vi "FGV_DataLoggerControl.vi"(7 "Actions":T1, 8 "Error In":errorcluster, 9 "Value":i32, 11 "VISA Refnum in":refnum<visa-resource-name>="COM1") -> (0 "Error Out":errorcluster, 1 "read buffer":string, 3 "VISA Refnum out":refnum<visa-resource-name>="COM1")   [LabVIEW 2014]
uses:
  Typedef_DataLogger_Actions.ctl
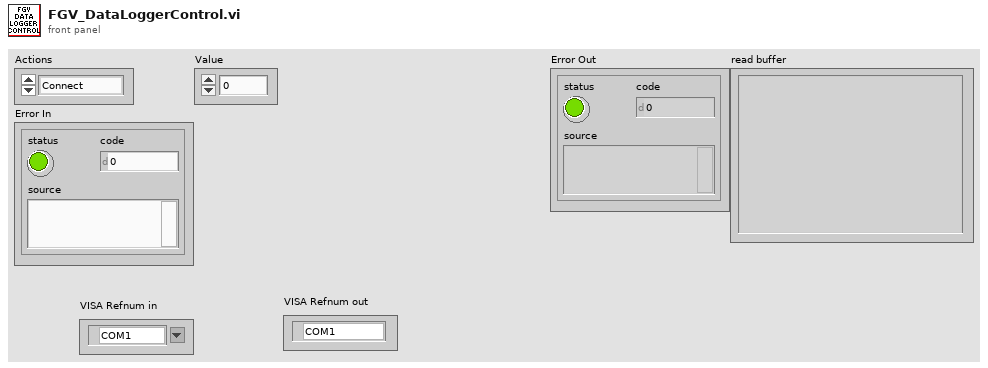
[diagram p1: front panel]
types:
  T1 = typedef "Typedef_DataLogger_Actions.ctl" = enum16{"Connect", "Disconnect", "Get Reading", "Set Offset", "Get Offset", "Set Time Step", "Get Time Step", "Save Settings", "Disable Readings", "Enable Readings"}
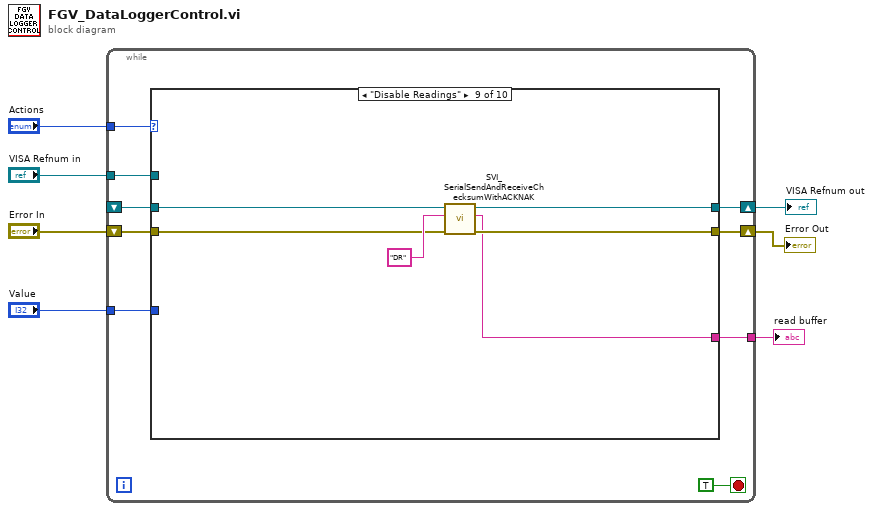
[diagram p0: block diagram]
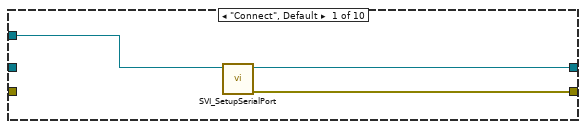
[diagram p2: hidden frame]
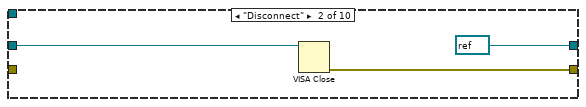
[diagram p3: hidden frame]
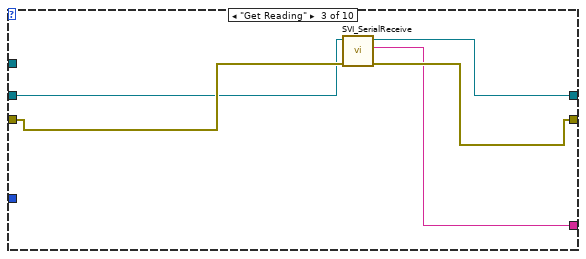
[diagram p4: hidden frame]
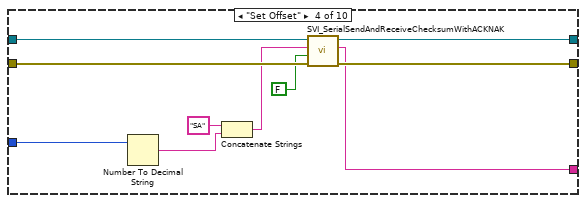
[diagram p5: hidden frame]
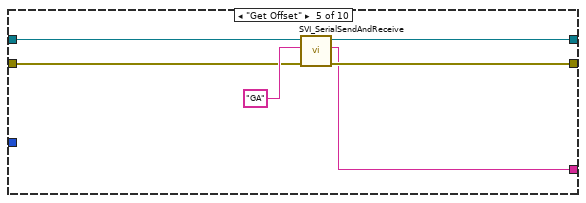
[diagram p6: hidden frame]
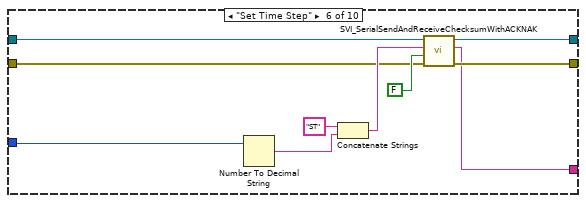
[diagram p7: hidden frame]
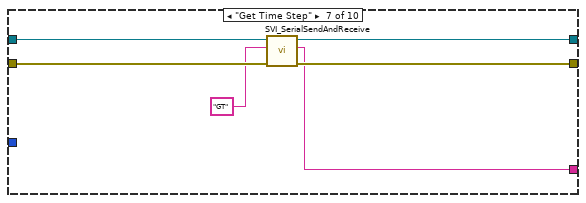
[diagram p8: hidden frame]
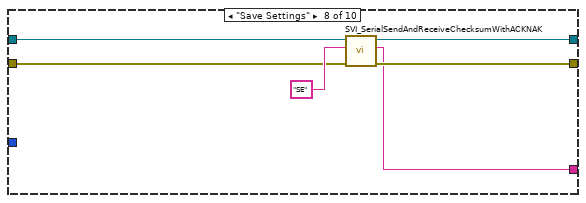
[diagram p9: hidden frame]
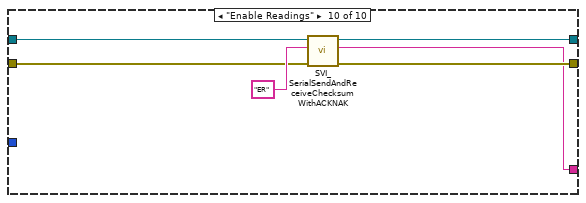
[diagram p10: hidden frame]
diagram:
  n1 = while {
    tunnel: "Actions" -> [w15]
    tunnel: "VISA Refnum in" -> [w14]
    shift-right: [w13] -> w3
    shift-left: _ -> [w11]
    shift-right: [w12] -> w5
    shift-left: "Error In" -> [w10]
    tunnel: "Value" -> [w9]
    tunnel: [w8] -> w1
    stop <- TRUE stop-if-true
    n2 = case shown="\"Disable Readings\"" w15 {
      tunnel: w14 -> [w19 _ _ _ _ _ _ _ _ _]
      tunnel: [w18 refnum<visa-resource-name> refnum ("VISA resource name out") w24 w33 w41 w46 w58 w63 w68 w74] -> w13
      tunnel: [w17 w22 w25 w34 w42 w47 w59 w64 w67 w73] -> w12
      tunnel: w11 -> [_ w20 w26 w36 w40 w48 w56 w62 w69 w75]
      tunnel: w10 -> [_ _ w27 w35 w39 w49 w57 w61 w70 w76]
      tunnel: w9 -> [_ _ _ w31 _ w45 _ _ _ _]
      tunnel: [_ _ w23 w28 w38 w44 w54 w60 w66 w72] -> w8
      frame "Connect", Default {
        n3 = call "SVI_SetupSerialPort.vi"("VISA Refnum in"=w19) -> ("error out"=w17:errorcluster, "VISA Refnum out"=w18:refnum<visa-resource-name>)  [unwired: 9 in]
      }
      frame "Disconnect" {
        n4 = VISA Close(VISA resource name=w20) -> (error out=w22:errorcluster)  [unwired: 1 in]
      }
      frame "Get Reading" {
        n5 = call "SVI_SerialReceive.vi"("error in (no error)"=w27, "VISA Refnum in"=w26) -> ("error out"=w25:errorcluster, "read buffer"=w23:string, "VISA resource name out"=w24:refnum<visa-resource-name>)  [unwired: 7 in]
      }
      frame "Set Offset" {
        n6 = Number To Decimal String(number=w31) -> (decimal integer string=w29:string)  [unwired: 1 in]
        n7 = Concatenate Strings("SA" ("Command"), w29) -> (w30:string)
        n8 = call "SVI_SerialSendAndReceiveChecksumWithACKNAK.vi"("error in (no error)"=w35, "Send Checksum"=FALSE, "Command"=w30, "VISA Refnum in"=w36) -> ("error out"=w34:errorcluster, "Received"=w28:string, "VISA resource name out"=w33:refnum<visa-resource-name>)  [unwired: 5 in]
      }
      frame "Get Offset" {
        n9 = call "SVI_SerialSendAndReceive.vi"("error in (no error)"=w39, "Command"="GA", "VISA Refnum in"=w40) -> ("error out"=w42:errorcluster, "read buffer"=w38:string, "VISA resource name out"=w41:refnum<visa-resource-name>)  [unwired: 6 in]
      }
      frame "Set Time Step" {
        n10 = Number To Decimal String(number=w45) -> (decimal integer string=w50:string)  [unwired: 1 in]
        n11 = Concatenate Strings("ST" ("Command"), w50) -> (w51:string)
        n12 = call "SVI_SerialSendAndReceiveChecksumWithACKNAK.vi"("error in (no error)"=w49, "Send Checksum"=FALSE, "Command"=w51, "VISA Refnum in"=w48) -> ("error out"=w47:errorcluster, "Received"=w44:string, "VISA resource name out"=w46:refnum<visa-resource-name>)  [unwired: 5 in]
      }
      frame "Get Time Step" {
        n13 = call "SVI_SerialSendAndReceive.vi"("error in (no error)"=w57, "Command"="GT", "VISA Refnum in"=w56) -> ("error out"=w59:errorcluster, "read buffer"=w54:string, "VISA resource name out"=w58:refnum<visa-resource-name>)  [unwired: 6 in]
      }
      frame "Save Settings" {
        n14 = call "SVI_SerialSendAndReceiveChecksumWithACKNAK.vi"("error in (no error)"=w61, "Command"="SE", "VISA Refnum in"=w62) -> ("error out"=w64:errorcluster, "Received"=w60:string, "VISA resource name out"=w63:refnum<visa-resource-name>)  [unwired: 6 in]
      }
      frame "Disable Readings" {
        n15 = call "SVI_SerialSendAndReceiveChecksumWithACKNAK.vi"("error in (no error)"=w70, "Command"="DR", "VISA Refnum in"=w69) -> ("error out"=w67:errorcluster, "Received"=w66:string, "VISA resource name out"=w68:refnum<visa-resource-name>)  [unwired: 6 in]
      }
      frame "Enable Readings" {
        n16 = call "SVI_SerialSendAndReceiveChecksumWithACKNAK.vi"("error in (no error)"=w76, "Command"="ER", "VISA Refnum in"=w75) -> ("error out"=w73:errorcluster, "Received"=w72:string, "VISA resource name out"=w74:refnum<visa-resource-name>)  [unwired: 6 in]
      }
    }
  }
  "VISA Refnum out" <- w3
  "Error Out" <- w5
  "read buffer" <- w1
